vi "Get Texture Data From Pointer.vi"(8 "error in (no error)":errorcluster, 11 "Surface Pointer":u32 format="%.0x") -> (0 "error out":errorcluster, 3 "Surface Data":T1 {"Blitmap Pointer" format="%.0x"; "Lock Data Pointer" format="%.0x"; "User Data Pointer" format="%.0x"; "Pixels Pointer" format="%.0x"; "Pixel Format Pointer" format="%.0x"})   [LabVIEW 2015]
uses:
  LibSDL2 Wrapper/Controls/Surface.ctl
  LibSDL2 Wrapper/Controls/Rectangle.ctl
  <vilib>/Utility/importsl/GetValueByPointer/datatype.ctl
  <vilib>/Utility/importsl/GetValueByPointer/GetValueByPointer.xnode
  LibSDL2 Wrapper/LibSDL2.lvlib
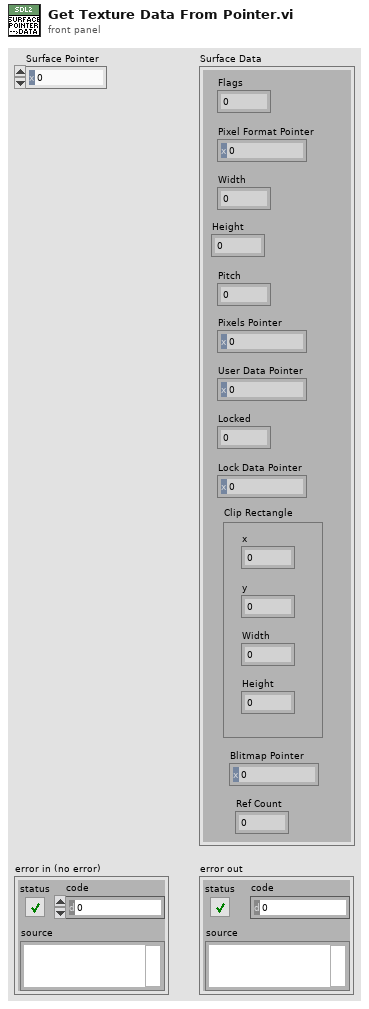
[diagram p1: front panel]
types:
  T1 = typedef "LibSDL2.lvlib/Surface.ctl" = cluster{"Flags":u32, "Pixel Format Pointer":u32, "Width":i32, "Height":i32, "Pitch":i32, "Pixels Pointer":u32, "User Data Pointer":u32, "Locked":i32, "Lock Data Pointer":u32, "Clip Rectangle":T2, "Blitmap Pointer":u32, "Ref Count":i32}
  T2 = typedef "LibSDL2.lvlib/Rectangle.ctl" = cluster{"x":i32, "y":i32, "Width":i32, "Height":i32}
  T3 = enum32{"pack1", "pack2", "pack4", "pack8", "pack16"}
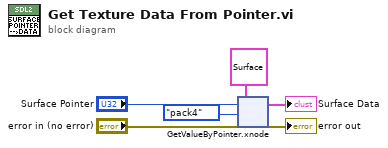
[diagram p0: block diagram]
diagram:
  n1 = xnode "GetValueByPointer.xnode"("Pointer"="Surface Pointer", "InputType"=T1 {"Flags"=0, "Pixel Format Pointer"=0, "Width"=0, "Height"=0, "Pitch"=0, "Pixels Pointer"=0, "User Data Pointer"=0, "Locked"=0, "Lock Data Pointer"=0, "Clip Rectangle"={"x"=0, "y"=0, "Width"=0, "Height"=0}, "Blitmap Pointer"=0, "Ref Count"=0} ("Surface"), "PackType"=T3."pack4", "ErrorIn"="error in (no error)") -> ("Output"=→"Surface Data":T1, "ErrorOut"=→"error out":errorcluster)
